vi "Read Waveform Measurement In Memory.vi"(5 "Destination Channel (1: Channel 2)":u16(ring)=1 items=["Channel 1", "Channel 2", "Channel 3", "Channel 4", "Math", "D0", "D1", "D2", "D3", "D4", "D5", "D6", "D7", "D8", "D9", "D10", "D11", "D12", "D13", "D14", "D15", "Reference 1", "Reference 2", "Reference 3", "Reference 4", "Amplitude", "Frequency", "Phase"], 6 "Measurement Number (0: Measurement 1)":i32(ring) items=["Measurement 1", "Measurement 2", "Measurement 3", "Measurement 4"], 7 "Measurement Function (21: Period)":i32(ring)=21 items=["Amplitude", "Area", "Burst Width", "Cycle Area", "Voltage Mean (cycle)", "Voltage RMS (cycle)", "Delay", "Fall Time", "Frequency", "Voltage High", "Voltage Low", "Voltage Max", "Voltage Mean", "Voltage Min", "Negative Duty Cycle", "Negative Edges Count", "Negative Overshoot", "Negative Pulses Count", "Negative Pulse Width", "Positive Duty Cycle", "Positive Edges Count", "Period", "Phase", "Vpp", "Positive Overshoot", "Positive Pulses Count", "Positive Pulse Width", "Rise Time", "Voltage RMS"], 8 "error in (no error)":errorcluster, 9 "Maximum Time (10000 ms)":u32=10000, 10 "Channel (0: Channel 1)":u16(ring) items=["Channel 1", "Channel 2", "Channel 3", "Channel 4", "Math", "D0", "D1", "D2", "D3", "D4", "D5", "D6", "D7", "D8", "D9", "D10", "D11", "D12", "D13", "D14", "D15", "Reference 1", "Reference 2", "Reference 3", "Reference 4", "Amplitude", "Frequency", "Phase"], 11 "VISA resource name":refnum<visa-resource-name>) -> (0 "error out":errorcluster, 2 "Measurement Value":dbl, 3 "VISA resource name out":refnum<visa-resource-name>)   [LabVIEW 2009, in "Tektronix DPO MSO 2000 4000 Series.lvlib"]
doc: "This VI invokes the <B>Fetch Displayed Waveform Measurement</B> VI to read the specified displayed measurement value.\n\nFirstly, initiates an acquisition on the channels that you enable with the <B>Configure Channel</B> VI. This VI then waits for the acquisition to complete, obtains a waveform measurement on the displayed measurement channel you specify, and returns the measurement value. The <B>Timeout</B> control specifies the maximum time to wait for operation complete in milliseconds.\n\n<B>Note:</B> \n\nYou must configure the appropriate reference levels before you call this VI.\n\nThe <B>Read Waveform Measurement</B> VI returns the immediate measurement (which is what is typically done) while this VI returns the specified displayed measurement.\n\nThis VI slows displayed measurements on the screen more than <B>Read Waveform Measurement</B> VI."
uses:
  <instrlib>/Tektronix DPO MSO 2000 4000 Series/Tektronix DPO MSO 2000 4000 Series.lvlib
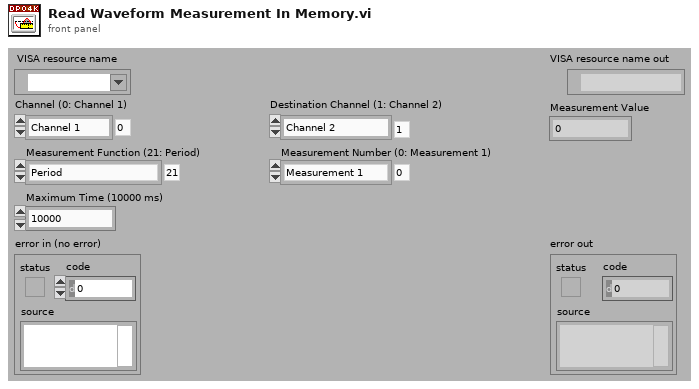
[diagram p1: front panel]
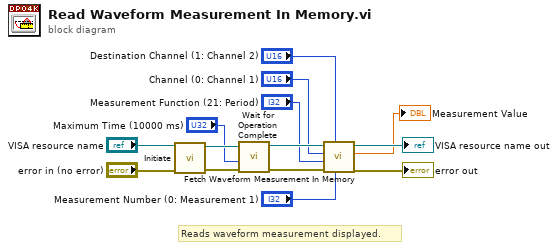
[diagram p0: block diagram]
diagram:
  # "Reads waveform measurement displayed."
  n1 = call <instrlib>:"Initiate.vi"("error in (no error)"="error in (no error)", "VISA resource name"="VISA resource name") -> ("error out"=w11:errorcluster, "VISA resource name out"=w12:refnum<visa-resource-name>)  [unwired: 8 in]
  n2 = call <instrlib>:"Wait for Operation Complete.vi"("error in (no error)"=w11, "Maximum Time (10000ms)"="Maximum Time (10000 ms)", "VISA resource name"=w12) -> ("error out"=w8:errorcluster, "VISA resource name out"=w9:refnum<visa-resource-name>)  [unwired: 7 in]
  n3 = call <instrlib>:"Fetch Waveform Measurement In Memory.vi"("Measurement Number (0: Measurement 1)"="Measurement Number (0: Measurement 1)", "Destination Channel (1: Channel 2)"="Destination Channel (1: Channel 2)", "error in (no error)"=w8, "Measurement Function (21: Period)"="Measurement Function (21: Period)", "Channel (0: Channel 1)"="Channel (0: Channel 1)", "VISA resource name"=w9) -> ("error out"=→"error out":errorcluster, "Measurement Value"=→"Measurement Value":dbl, "VISA resource name out"=→"VISA resource name out":refnum<visa-resource-name>)  [unwired: 3 in]
